vi "x-axis.vi"(8 "error in (no error)":errorcluster, 11 "Wavelength in":refnum<class "Wavelength Triax 550.lvclass">) -> (0 "error out":errorcluster, 1 "Label":string, 2 "Unit":string, 3 "Wavelength out":refnum<class "Wavelength Triax 550.lvclass">)   [LabVIEW 2017, in "Wavelength Triax 550.lvclass"]
uses:
  Wavelength Triax 550.lvclass
  Scanner/Scanner.lvclass
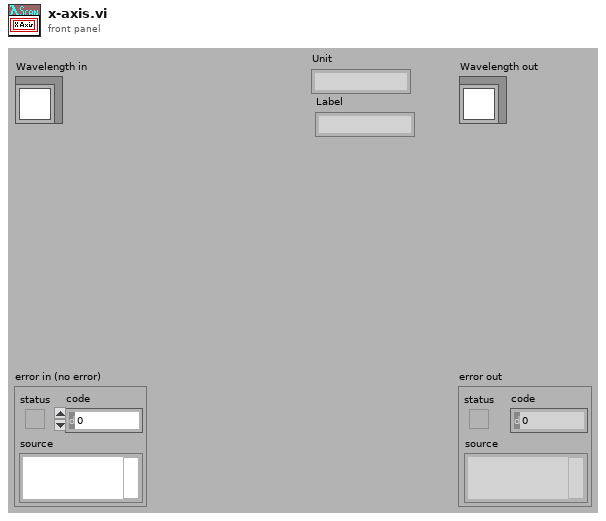
[diagram p1: front panel]
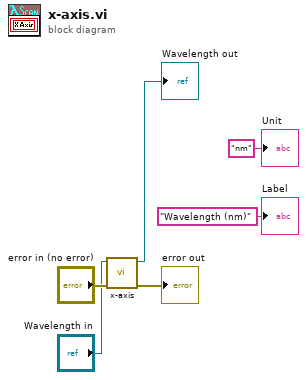
[diagram p0: block diagram]
diagram:
  n1 = call-parent "x-axis.vi"("error in (no error)"="error in (no error)", "Scanner in"="Wavelength in") -> ("error out"=→"error out":errorcluster, "Scanner out"=→"Wavelength out":refnum<class "Wavelength Triax 550.lvclass">)  [unwired: 6 in, 2 out]
  "Label" <- "Wavelength (nm)" ("Label")
  "Unit" <- "nm" ("Unit")
